vi "Schedule.Write.vi"(8 "error in (no error)":errorcluster, 10 "Data to Write":variant, 11 "Schedule <JSON> In":string="{}") -> (0 "error out":errorcluster, 3 "Schedule <JSON> Out":string="{}")   [LabVIEW 2019, in "ObjectSettings.lvclass"]
uses:
  ObjectSettings.lvclass
  585efb58-4a7b-4046-b048-a95b4228d0b9.vi
  <vilib>/JDP Science/JSONtext/Variant to JSON Text.vi
  <vilib>/JDP Science/JSONtext/LVClass Serializer/JSONtext LVClass Serializer.lvclass
  <vilib>/JDP Science/JSONtext/JSONtext.lvlib
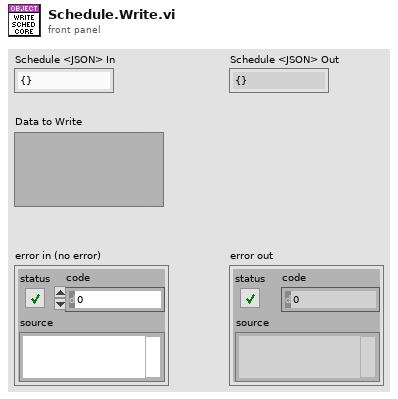
[diagram p1: front panel]
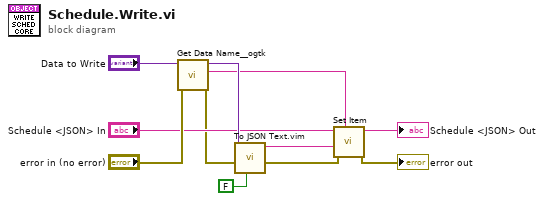
[diagram p0: block diagram]
diagram:
  n1 = call <userlib>:"Get Data Name__ogtk.vi"("error in (no error)"="error in (no error)", "Data"="Data to Write") -> ("error out"=w2:errorcluster, "Data Name"=w4:string, "Data dup"=w10:variant)  [unwired: 7 in]
  n2 = call "To JSON Text.vim"("Pretty Print?"=FALSE, "error in (no error)"=w2, "Anything"=w10) -> ("error out"=w1:errorcluster, "<JSON>"=w3:string)  [unwired: 7 in]
  n3 = call <vilib>:"Set Item.vi"("$Path or Item Name"=w4, "error in (no error)"=w1, "JSON to Insert"=w3, "JSON"="Schedule <JSON> In") -> ("error out"=→"error out":errorcluster, "<JSON>"=→"Schedule <JSON> Out":string)  [unwired: 4 in, 1 out]
